vi "Teleop - Turbo Turn Reduce (SubVI).vi"(9 "Turbo":bool, 10 "Right Drive in":dbl, 11 "Left Drive in":dbl) -> (2 "Right Drive out":dbl, 3 "Left Drive out":dbl)   [LabVIEW 2019]
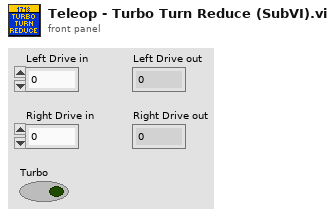
[diagram p1: front panel]
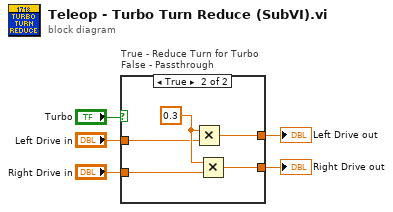
[diagram p0: block diagram]
diagram:
  n1 = case "True - Reduce Turn for Turbo\nFalse - Passthrough" shown="True" "Turbo" {
    tunnel: [w7 w8] -> w2
    tunnel: "Left Drive in" -> [w7 w9]
    tunnel: "Right Drive in" -> [w6 w11]
    tunnel: [w6 w10] -> w4
    frame False {
    }
    frame True {
      w12 = 0.3 ("x")
      n2 = Multiply(x=w12, y=w9) -> (x*y=w8:dbl)
      n3 = Multiply(x=w12, y=w11) -> (x*y=w10:dbl)
    }
  }
  "Right Drive out" <- w4
  "Left Drive out" <- w2
